vi "AMI1.vi"() -> ()   [LabVIEW 2013]
panel:
  out "AMI码波形图":dbl[](graph)
  in  "停止":bool
  in  "计数":u8
  out "变换后的AM码":i8[](array[numeric])
  in  "原消息代码":u32[](array[numeric])
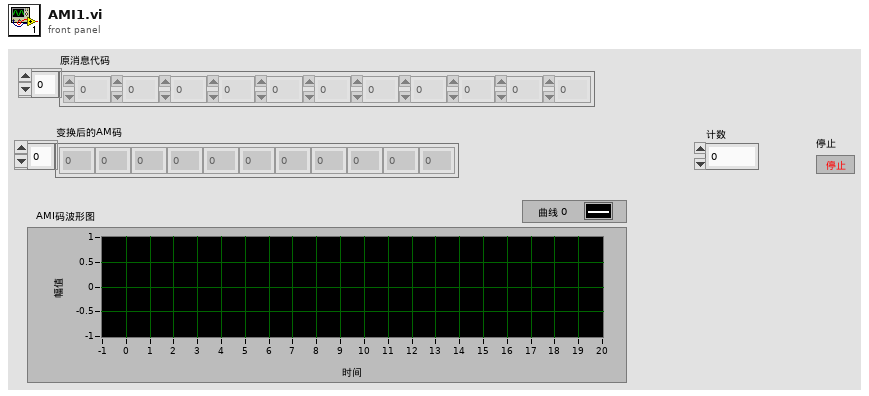
[diagram p1: front panel]
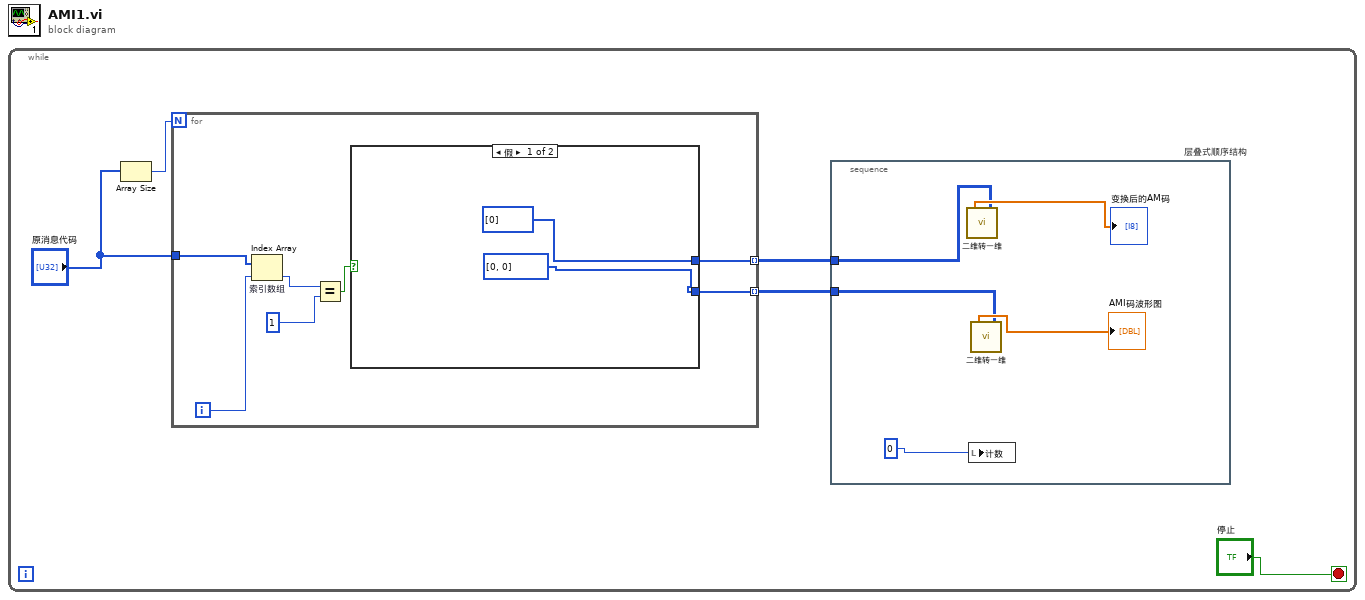
[diagram p0: block diagram]
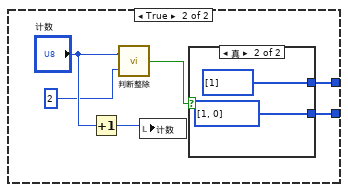
[diagram p2: hidden frame]
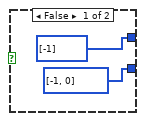
[diagram p3: hidden frame]
diagram:
  n1 = while {
    stop <- "停止" stop-if-true
    n2 = Array Size(array="原消息代码") -> (size(s)=w2:i32)
    n3 = for {
      N: w2 -> [_]
      tunnel: [w17] -> w4 mode=indexing
      tunnel: [w16] -> w3 mode=indexing
      tunnel: "原消息代码" -> [w14]
      i -> [w13]
      n4 = Index Array "索引数组"(array=w14, index=w13) -> (element=w12:u32)
      n5 = Equal?(x=w12, y=1) -> (x = y?=w15:bool)
      n6 = case shown="假" w15 {
        tunnel: [i32[] [0] w21] -> w17
        tunnel: [i32[] [0, 0] w20] -> w16
        frame False {
        }
        frame True {
          n7 = Increment(x="计数") -> (x+1=w22:u8)
          n8 = call "判断整除.vi"("被除数"=2, "除数"="计数") -> ("布尔"=w23:bool)
          n9 = local write "计数"(w22) -> ()
          n10 = case shown="真" w23 {
            tunnel: [i32[] [-1] i32[] [1]] -> w21
            tunnel: [i32[] [-1, 0] i32[] [1, 0]] -> w20
            frame False {
            }
            frame True {
            }
          }
        }
      }
    }
    n11 = stacked-sequence "层叠式顺序结构" {
      tunnel: w4 -> [w7]
      tunnel: w3 -> [w6]
      frame #0 {
        n12 = call "二维转一维.vi"("输入2维"=w7) -> ("输出一维"=→"变换后的AM码":dbl[])
        n13 = local write "计数"(0) -> ()
        n14 = call "二维转一维.vi"("输入2维"=w6) -> ("输出一维"=→"AMI码波形图":dbl[])
      }
    }
  }
